vi "CPP_SpectraFit.vi"() -> (5 "Plug in titles":string[](array[string]), 7 "Plug in values":string[](array[string]))   [LabVIEW 2011]
uses:
  Controls/Instrument_Array.ctl
  Controls/Post_Process.ctl
  Controls/Graph_Type.ctl
  Globals/Meas_global.vi
  Globals/Plug_in_data_global.vi
panel:
  in  "Divider":i32(slide)=10 scale=1.0..100000.0 scale format="%#_6e"
  out "dF/ Hz":dbl
  in  "Show Smooth":bool=TRUE
  in  "Save Spectra?":bool
  in  "Desired number of samples per block":i32=32768
  out "Spectra":cluster{"Frequencies":dbl[], dbl[]}[](graph)
  in  "Averaging samples":i32=1 min=1 max=1000
  in  "Spectra Index (from ALL channels)":i32
  out "Waveform Graph":dbl[][](graph)
  in  "Channels to Plot":i32[](array[ring])=[0] items=["Pitot (Uref)", "HW (Uhw)", "Save Nothing"]
  # "Run this VI to update the channel names"
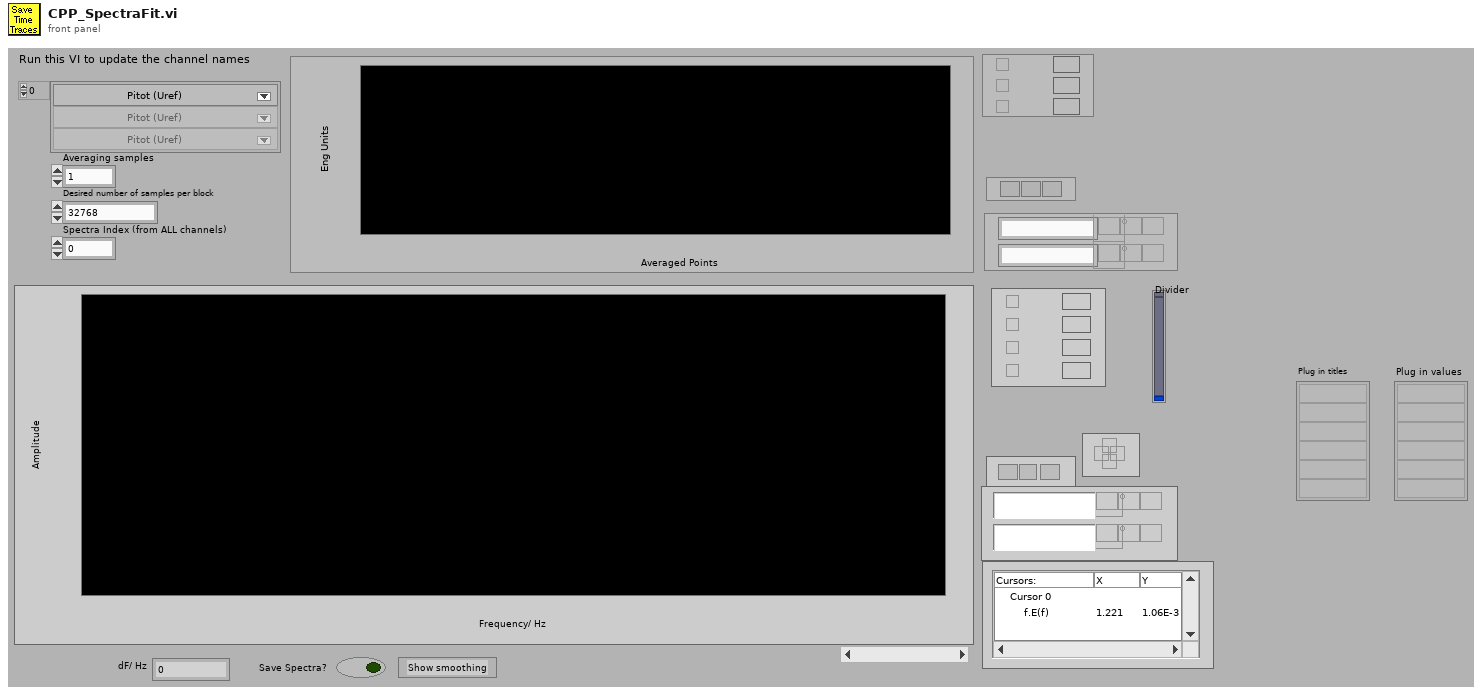
[diagram p1: front panel]
types:
  T1 = typedef "Analysis_info_cluster.ctl" = cluster{"Colour":u32, "Inst type":T2, "Inst name":string, "Symbol":string, "Code name":string, "Extra Info":string, "Inst Array":T3, "Index":i32, "Voltage Index":i32, "Extra Titles":string[], "Extra Values":string[]}
  T2 = typedef "Inst_type.ctl" = enum16{"Propeller anemometer", "Raw voltage", "Pressure Transducer", "Pitot-static tube", "Preston tube", "Hot wire", "Cross wire 1", "Cross wire 2", "Generic Linear", "Generic Polynomial", "Generic BackPoly", "Fast FID", "Thermocouple", "Cold wire", "Pulsed Wire", "LDA Vel", "LDA Tran time", "LDA Arr time"}
  T3 = typedef "Instrument_Array.ctl" = enum16{"PWA", "LDA", "Analogue"}
  T4 = typedef "Post_Process.ctl" = enum16{"Take New Data", "Post Process Raw Data File"}
  T5 = typedef "Graph_Type.ctl" = enum16{"Show no graph", "Voltage trace", "Velocity trace", "Vel histogram", "Spectrum", "f.E(f) v Log f", "Auto-Corr"}
  T6 = cluster{"Plot 1":u16, "Plot 2":u16, "Save graph":u16, "Plot Type":T5}
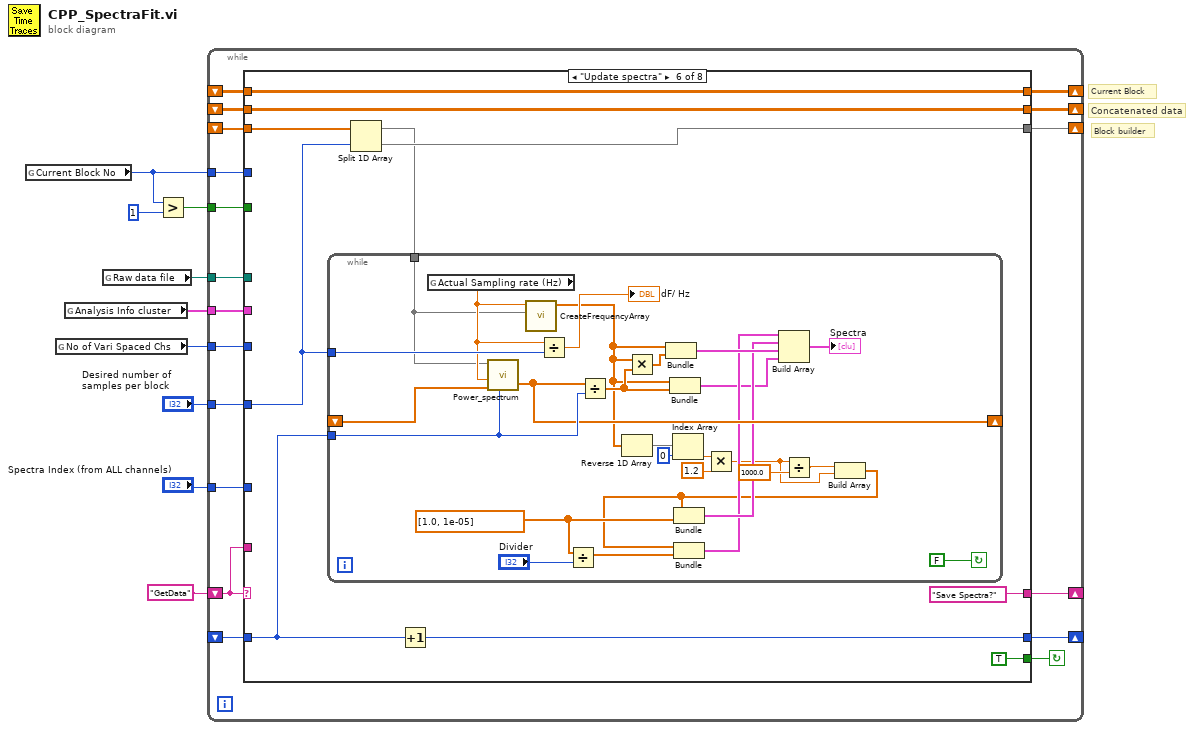
[diagram p0: block diagram]
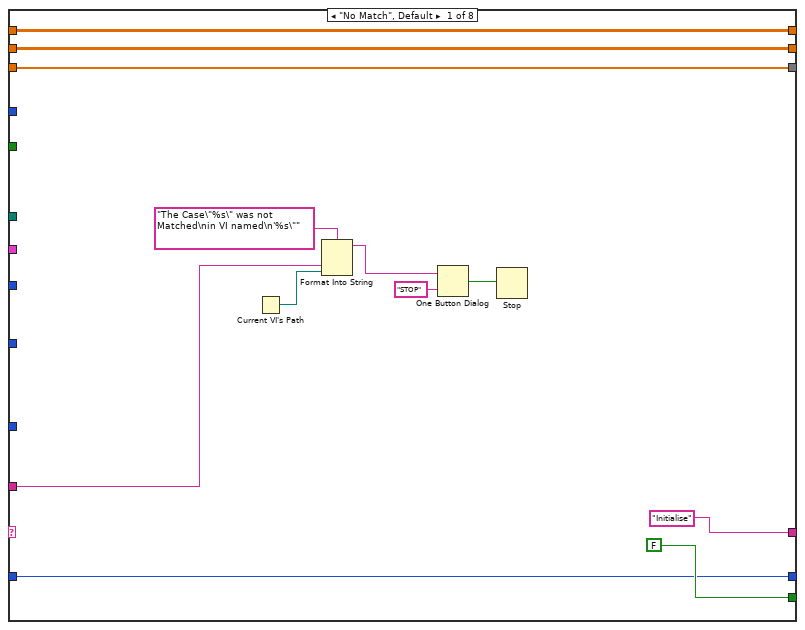
[diagram p2: hidden frame]
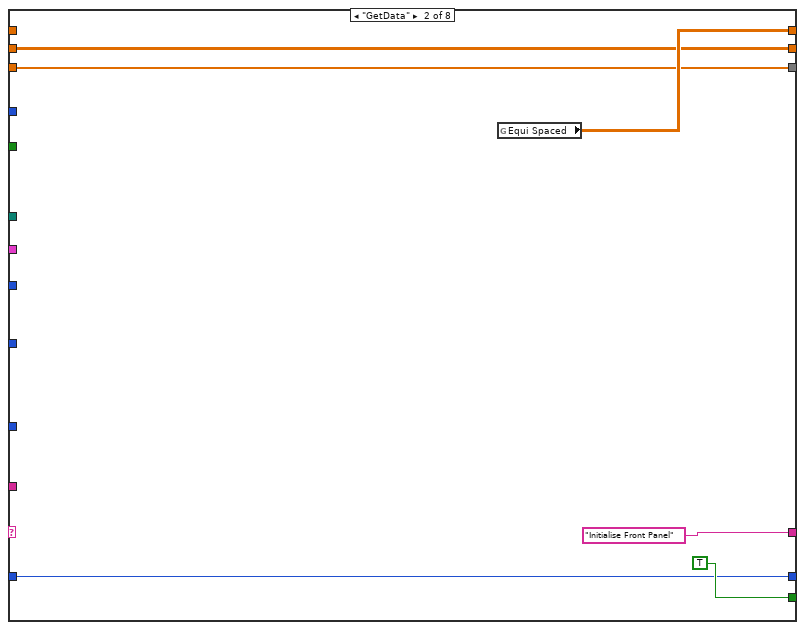
[diagram p3: hidden frame]
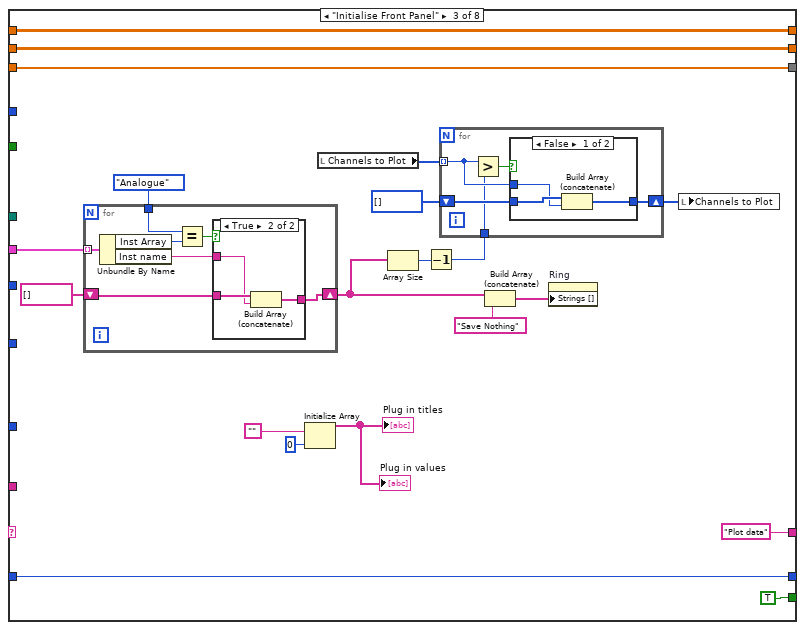
[diagram p4: hidden frame]
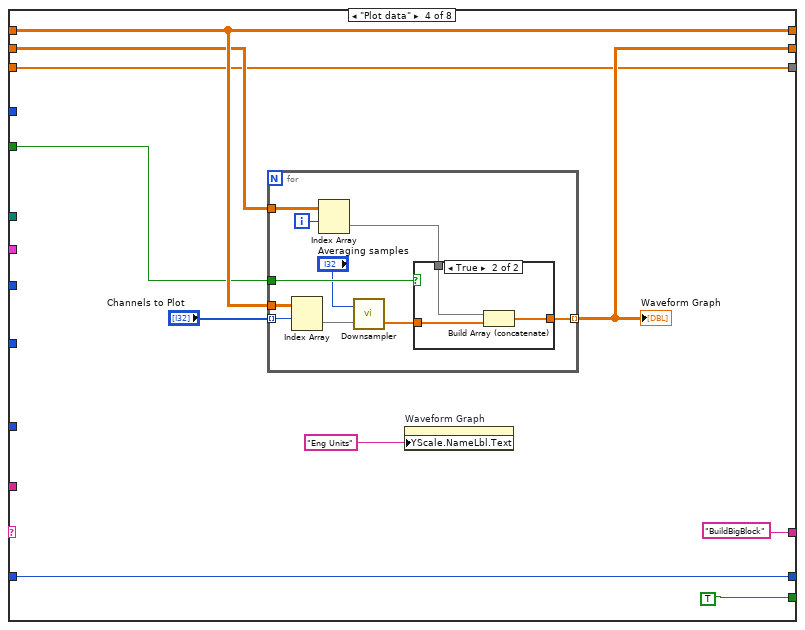
[diagram p7: hidden frame]
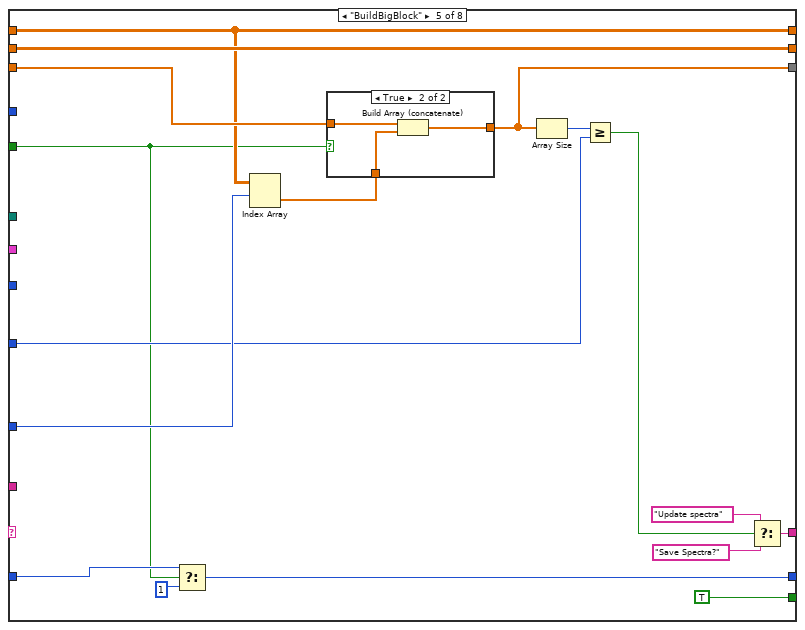
[diagram p9: hidden frame]
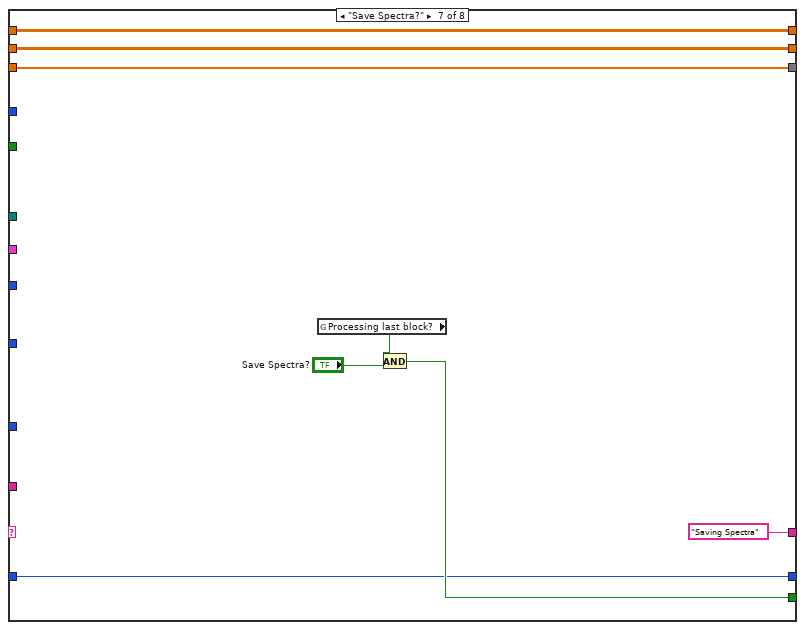
[diagram p11: hidden frame]
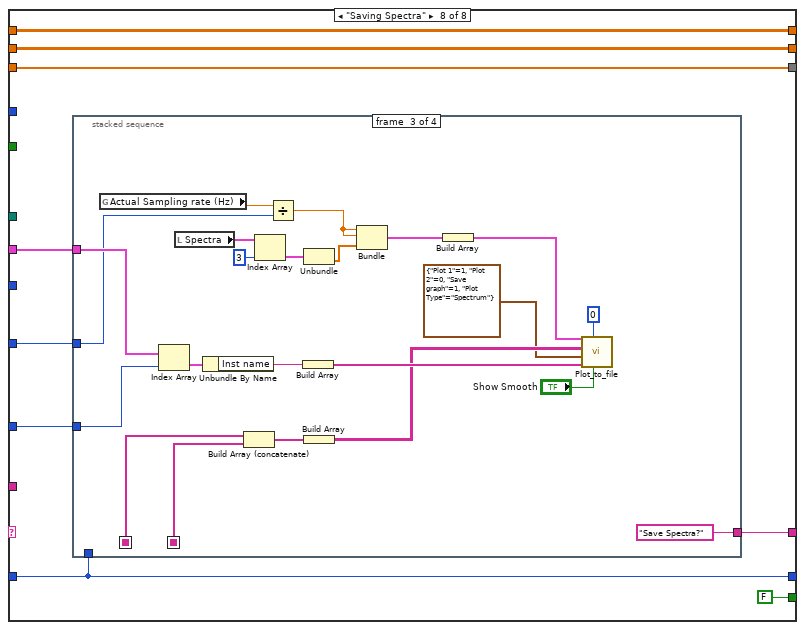
[diagram p12: hidden frame]
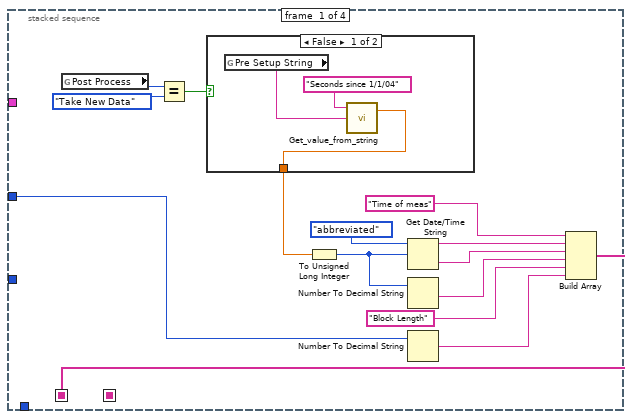
[diagram p13: hidden frame]
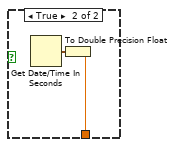
[diagram p14: hidden frame]
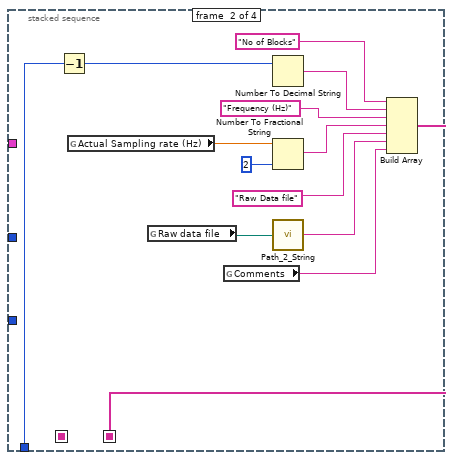
[diagram p15: hidden frame]
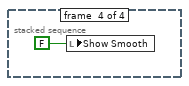
[diagram p16: hidden frame]
diagram:
  # "Block builder"
  # "Concatenated data"
  # "Current Block"
  n1 = global read "Meas_global.vi" "Current Block No"() -> (w6:i32)
  n2 = global read "Meas_global.vi" "No of Vari Spaced Chs"() -> (w4:i32)
  n3 = global read "Meas_global.vi" "Analysis Info cluster"() -> (w5:T1[])
  n4 = global read "Meas_global.vi" "Raw data file"() -> (w8:path)
  n5 = Greater?(x=w6, y=1) -> (0:w3:bool)
  n6 = while {
    shift-left: "GetData" -> [w25]
    shift-right: [w26] -> _
    tunnel: w8 -> [w24]
    tunnel: w3 -> [w23]
    tunnel: w6 -> [w22]
    tunnel: w5 -> [w21]
    tunnel: w4 -> [w20]
    shift-right: [w19] -> _
    shift-left: _ -> [w18]
    shift-right: [w16] -> _
    shift-left: _ -> [w17]
    shift-right: [w14] -> _
    shift-left: _ -> [w15]
    tunnel: "Desired number of samples per block" -> [w13]
    tunnel: "Spectra Index (from ALL channels)" -> [w12]
    shift-right: [w11] -> _
    shift-left: _ -> [w10]
    stop <- w27 continue-if-true
    n7 = case shown="\"Update spectra\"" w25 {
      tunnel: [FALSE TRUE TRUE TRUE ("Calculate Spectra and Histogram?") TRUE ("Calculate Spectra and Histogram?") TRUE ("Calculate Spectra and Histogram?") w169 FALSE ("Calculate Spectra and Histogram?")] -> w27
      tunnel: ["Initialise" "Initialise Front Panel" "Plot data" "BuildBigBlock" ("t") w111 "Save Spectra?" "Saving Spectra" w182] -> w26
      tunnel: w25 -> [w34 _ _ _ _ _ _ _]
      tunnel: w24 -> [_ _ _ _ _ _ _ _]
      tunnel: w23 -> [_ _ _ w93 w114 _ _ _]
      tunnel: w22 -> [_ _ _ _ _ _ _ _]
      tunnel: w21 -> [_ _ w49 _ _ _ _ w180]
      tunnel: w20 -> [_ _ _ _ _ _ _ _]
      tunnel: [w31 w43 w55 w95 w124 w139 w174 w183] -> w19
      tunnel: w18 -> [w31 _ w55 w95 w124 w139 w174 w183]
      tunnel: w17 -> [w30 w42 w54 w94 w125 w140 w175 w184]
      tunnel: [w30 w42 w54 w91 w125 w140 w175 w184] -> w16
      tunnel: w15 -> [w29 w41 w51 w89 w126 w138 w172 w181]
      tunnel: [w29 w41 w51 w89 w122 w137 w172 w181] -> w14
      tunnel: w13 -> [_ _ _ _ w118 w133 _ w177]
      tunnel: w12 -> [_ _ _ _ w120 _ _ w179]
      tunnel: [w28 w40 w50 w88 w115 w131 w168 w176] -> w11
      tunnel: w10 -> [w28 w40 w50 w88 w116 w132 w168 w176]
      frame "No Match", Default {
        n8 = Current VI's Path() -> (path=w33:path)
        n9 = Format Into String(format string="The Case\"%s\" was not Matched\nin VI named\n'%s\"" ("Format String"), w34, w33) -> (resulting string=w37:string)  [unwired: 2 in, 1 out]
        n10 = One Button Dialog(message=w37, button name ("OK")="STOP") -> (true=w35:bool)
        n11 = Stop(stop? (T)=w35) -> ()
      }
      frame "GetData" {
        n12 = global read "Plug_in_data_global.vi" "Equi Spaced"() -> (w43:dbl[][])
      }
      frame "Initialise Front Panel" {
        n13 = for {
          tunnel: Instrument_Array."Analogue" ("Inst Array") -> [w71]
          tunnel: w49 -> [w70] mode=indexing
          shift-right: [w67] -> w48
          shift-left: string[] [] -> [w68]
          n14 = Unbundle By Name(w70) -> ("Inst Array"=w72:T3, "Inst name"=w66:string)
          n15 = Equal?(x=w71, y=w72) -> (x = y?=w69:bool)
          n16 = case shown="True" w69 {
            tunnel: w68 -> [w73 w76]
            tunnel: [w73 w75] -> w67
            tunnel: w66 -> [_ w74]
            frame False {
            }
            frame True {
              n17 = Build Array (concatenate)(w76, w74) -> (w75:string[])
            }
          }
        }
        n18 = Initialize Array("", 0) -> (→"Plug in values" →"Plug in titles":string[])
        n19 = local read "Channels to Plot"() -> (w62:i32[])
        n20 = Array Size(array=w48) -> (size(s)=w57:i32)
        n21 = Decrement(x=w57) -> (x-1=w56:i32)
        n22 = for {
          tunnel: w62 -> [w78] mode=indexing
          shift-right: [w79] -> w60
          shift-left: i32[] [] -> [w80]
          tunnel: w56 -> [w77]
          n23 = Greater?(x=w78, y=w77) -> (0:w81:bool)
          n24 = case shown="False" w81 {
            tunnel: w80 -> [w84 w85]
            tunnel: [w83 w85] -> w79
            tunnel: w78 -> [w82 _]
            frame False {
              n25 = Build Array (concatenate)(w84, w82) -> (w83:i32[])
            }
            frame True {
            }
          }
        }
        n26 = Build Array (concatenate)(w48, "Save Nothing") -> (w58:string[])
        n27 = property on="Ring" class="Ring (strict)"("Strings []"=w58) -> ()  [unwired: 2 in, 2 out]
        n28 = local write "Channels to Plot"(w60) -> ()
      }
      frame "Plot data" {
        n29 = for {
          tunnel: w95 -> [w105]
          tunnel: "Channels to Plot" -> [w104] mode=indexing
          tunnel: w94 -> [w101]
          tunnel: [w102] -> w91 mode=indexing
          tunnel: w93 -> [w103]
          i -> [w100]
          n30 = Index Array(array=w105, index (row)=w104) -> (element=w98:dbl[])  [unwired: 1 in]
          n31 = Index Array(array=w101, index (row)=w100) -> (element=w99:dbl[])  [unwired: 1 in]
          n32 = call "Downsampler.vi"("Input Array"=w98, "Averaging samples"="Averaging samples") -> ("Downsampled Array"=w97:dbl[])  [unwired: 1 out]
          n33 = case shown="True" w103 {
            tunnel: w99 -> [_ w109]
            tunnel: w97 -> [w106 w108]
            tunnel: [w106 w107] -> w102
            frame False {
            }
            frame True {
              n34 = Build Array (concatenate)(w109, w108) -> (w107:dbl[])
            }
          }
        }
        "Waveform Graph" <- w91
        n35 = property on="Waveform Graph" class="WFGraph (strict)"("YScale.NameLbl.Text"="Eng Units") -> ()  [unwired: 2 in, 2 out]
      }
      frame "BuildBigBlock" {
        n36 = Select(t=w116, s=w114, f=1) -> (s? t:f=w115:i32)
        n37 = Index Array(array=w124, index (row)=w120) -> (element=w123:dbl[])  [unwired: 1 in]
        n38 = case shown="True" w114 {
          tunnel: w126 -> [_ w130]
          tunnel: [w127 w129] -> w122
          tunnel: w123 -> [w127 w128]
          frame False {
          }
          frame True {
            n39 = Build Array (concatenate)(w130, w128) -> (w129:dbl[])
          }
        }
        n40 = Array Size(array=w122) -> (size(s)=w121:i32)
        n41 = Greater Or Equal?(x=w121, y=w118) -> (x >= y?=w110:bool)
        n42 = Select(t="Update spectra", s=w110, f="Save Spectra?") -> (s? t:f=w111:string)
      }
      frame "Update spectra" {
        n43 = Split 1D Array(array=w138, index=w133) -> (first subarray=w134:dbl[], second subarray=w137:dbl[])
        n44 = while {
          shift-left: _ -> [w162]
          shift-right: [w163] -> _
          tunnel: w134 -> [w160]
          tunnel: w132 -> [w166]
          tunnel: w133 -> [w165]
          stop <- FALSE continue-if-true
          w155 = dbl[] [1.0, 1e-05]
          n45 = global read "Meas_global.vi" "Actual Sampling rate (Hz)"() -> (w161:dbl)
          n46 = call "Power_spectrum.vi"("U"=w160, "Sampling frequency"=w161, "Spectrum input array"=w162, "Block No"=w166) -> ("Spectrum output array"=w163:dbl[])  [unwired: 1 in, 1 out]
          n47 = call "CreateFrequencyArray.vi"("Signal"=w160, "Actual Sampling rate (Hz)"=w161) -> ("Frequencies"=w149:dbl[])  [unwired: 9 in]
          n48 = Divide(x=w161, y=w165) -> (x/y=→"dF/ Hz":dbl)
          n49 = Divide(x=w155, y="Divider") -> (x/y=w156:dbl[])
          n50 = Divide(x=w163, y=w166) -> (x/y=w151:dbl[])
          n51 = Reverse 1D Array(array=w149) -> (reversed array=w148:dbl[])
          n52 = Multiply(x=w149, y=w151) -> (x*y=w152:dbl[])
          n53 = Bundle("Frequencies"=w149, w152) -> (w158:cluster{"Frequencies":dbl[], dbl[]})  [unwired: 1 in]
          n54 = Bundle("Frequencies"=w149, w151) -> (w150:cluster{"Frequencies":dbl[], dbl[]})  [unwired: 1 in]
          n55 = Index Array(array=w148, index=0) -> (element=w146:dbl)
          n56 = Multiply(x=w146, y=1.2) -> (x*y=w142:dbl)
          n57 = Divide(x=w142, y=1000.0) -> (x/y=w143:dbl)
          n58 = Build Array(w143, w142) -> (w141:dbl[])
          n59 = Bundle(w141, w155) -> (w157:cluster{dbl[], dbl[]})  [unwired: 1 in]
          n60 = Bundle(w141, w156) -> (w153:cluster{dbl[], dbl[]})  [unwired: 1 in]
          n61 = Build Array(w153, w157, w158, w150) -> (→"Spectra":cluster{"Frequencies":dbl[], dbl[]}[])
        }
        n62 = Increment(x=w132) -> (x+1=w131:i32)
      }
      frame "Save Spectra?" {
        n63 = global read "Meas_global.vi" "Processing last block?"() -> (w170:bool)
        n64 = And(x=w170, y="Save Spectra?") -> (x .and. y?=w169:bool)
      }
      frame "Saving Spectra" {
        n65 = stacked-sequence {
          seq-local: [w188 _ _ _] -> [_ _ w230 _]
          seq-local: [_ w208 _ _] -> [_ _ w229 _]
          tunnel: [_ _ "Save Spectra?" _] -> w182
          tunnel: w180 -> [_ _ w236 _]
          tunnel: w179 -> [_ _ w235 _]
          tunnel: w177 -> [w186 _ w221 _]
          tunnel: w176 -> [_ w206 _ _]
          frame #0 {
            n66 = global read "Meas_global.vi" "Post Process"() -> (w190:T4)
            n67 = Equal?(x=w190, y=Post_Process."Take New Data" ("Post Process")) -> (x = y?=w191:bool)
            n68 = case shown="False" w191 {
              tunnel: [w199 w203] -> w192
              frame False {
                n69 = global read "Meas_global.vi" "Pre Setup String"() -> (w200:string)
                n70 = call "Get_value_from_string.vi"("Input string"=w200, "Variable name"="Seconds since 1/1/04") -> ("Value"=w199:dbl)  [unwired: 1 in, 1 out]
              }
              frame True {
                n71 = Get Date/Time In Seconds() -> (seconds since 1Jan1904=w202:timestamp)
                n72 = To Double Precision Float(number=w202) -> (double precision float=w203:dbl)
              }
            }
            n73 = To Unsigned Long Integer(number=w192) -> (unsigned 32bit integer=w196:u32)
            n74 = Get Date/Time String(date format (0)=enum16{"short", "long", "abbreviated"}."abbreviated", seconds (now)=w196) -> (date string=w194:string, time string=w195:string)  [unwired: 1 out]
            n75 = Number To Decimal String(number=w196) -> (decimal integer string=w197:string)  [unwired: 1 out]
            n76 = Number To Decimal String(number=w186) -> (decimal integer string=w185:string)  [unwired: 1 out]
            n77 = Build Array("Time of meas", w194, w195, w197, "Block Length" ("element"), w185) -> (w188:string[])
          }
          frame #1 {
            n78 = Decrement(x=w206) -> (x-1=w205:i32)
            n79 = global read "Meas_global.vi" "Actual Sampling rate (Hz)"() -> (w209:dbl)
            n80 = global read "Meas_global.vi" "Raw data file"() -> (w215:path)
            n81 = global read "Meas_global.vi" "Comments"() -> (w214:string)
            n82 = Number To Decimal String(number=w205) -> (decimal integer string=w204:string)  [unwired: 1 out]
            n83 = Number To Fractional String(number=w209, precision (6)=i16 2) -> (F-format string=w212:string)  [unwired: 2 out]
            n84 = call "Path_2_String.vi"("Real Path"=w215) -> ("Path String"=w216:string)
            n85 = Build Array("No of Blocks", w204, "Frequency (Hz)", w212, "Raw Data file", w216, w214) -> (w208:string[])
          }
          frame #2 {
            n86 = global read "Meas_global.vi" "Actual Sampling rate (Hz)"() -> (w222:dbl)
            n87 = Index Array(array=w236, index=w235) -> (element=w234:T1)
            n88 = local read "Spectra"() -> (w225:cluster{"Frequencies":dbl[], dbl[]}[])
            n89 = Unbundle By Name(w234) -> ("Inst name"=w233:string)
            n90 = Build Array (concatenate)(w230, w229) -> (w228:string[])
            n91 = Index Array(array=w225, index=3) -> (element=w223:cluster{"Frequencies":dbl[], dbl[]})
            n92 = Divide(x=w222, y=w221) -> (x/y=w219:dbl)
            n93 = Build Array(w233) -> (w232:string[])
            n94 = Unbundle(w223) -> (w220:dbl[])  [unwired: 1 out]
            n95 = Build Array(w228) -> (w227:string[][])
            n96 = Bundle(w219, w219, w220) -> (w218:cluster{dbl, dbl, dbl[]})  [unwired: 1 in]
            n97 = Build Array(w218) -> (w217:cluster{dbl, dbl, dbl[]}[])
            n98 = call "Plot_to_file.vi"("Show Smooth"="Show Smooth", "Start trace No"=0, "Trace names"=w232, "Graph"=T6 {"Plot 1"=1, "Plot 2"=0, "Save graph"=1, "Plot Type"=enum."Spectrum"}, "Plot file label"=w227, "Plot data"=w217) -> ()  [unwired: 6 out]
          }
          frame #3 {
            n99 = local write "Show Smooth"(FALSE ("Show Smooth")) -> ()
          }
        }
      }
    }
  }
